vi "TagEvent.vi"(8 "error in":errorcluster, 9 "Acquisition mode in":T8, 11 "Processing loop vars in":T1 {"CurrInverter"."last updated" format="%<%H:%M\n%d/%m/%Y>T"; "CurrInverter"."set flag" items=["False", "True"]}) -> (0 "error out":errorcluster, 3 "Processing loop vars out":T1 {"CurrInverter"."last updated" format="%<%H:%M\n%d/%m/%Y>T"; "CurrInverter"."set flag" items=["False", "True"]})   [LabVIEW 2019, in "Main.lvclass"]
uses:
  Main.lvclass
  DataTypes/averaging variables.ctl
  DataTypes/ESR alarm variables.ctl
  Common/DataTypes/inverter gain range--cluster.ctl
  Common/DataTypes/inverter offset range--cluster.ctl
  Common/DataTypes/inverter info v2--cluster.ctl
  Common/DataTypes/Inverter database record v2--cluster.ctl
  DataTypes/Processing loop variables--cluster.ctl
  Common/DataTypes/Acquisition Mode--cluster.ctl
panel:
  out "Current Tag Event":i32
  out "Step Up":dbl
  out "Start time":dbl
  out "Time difference":i32
  out "Current seconds":dbl
  out "Step Down":dbl
  out "Calculated Total Power":dbl
  out "Calculated Local Power":dbl
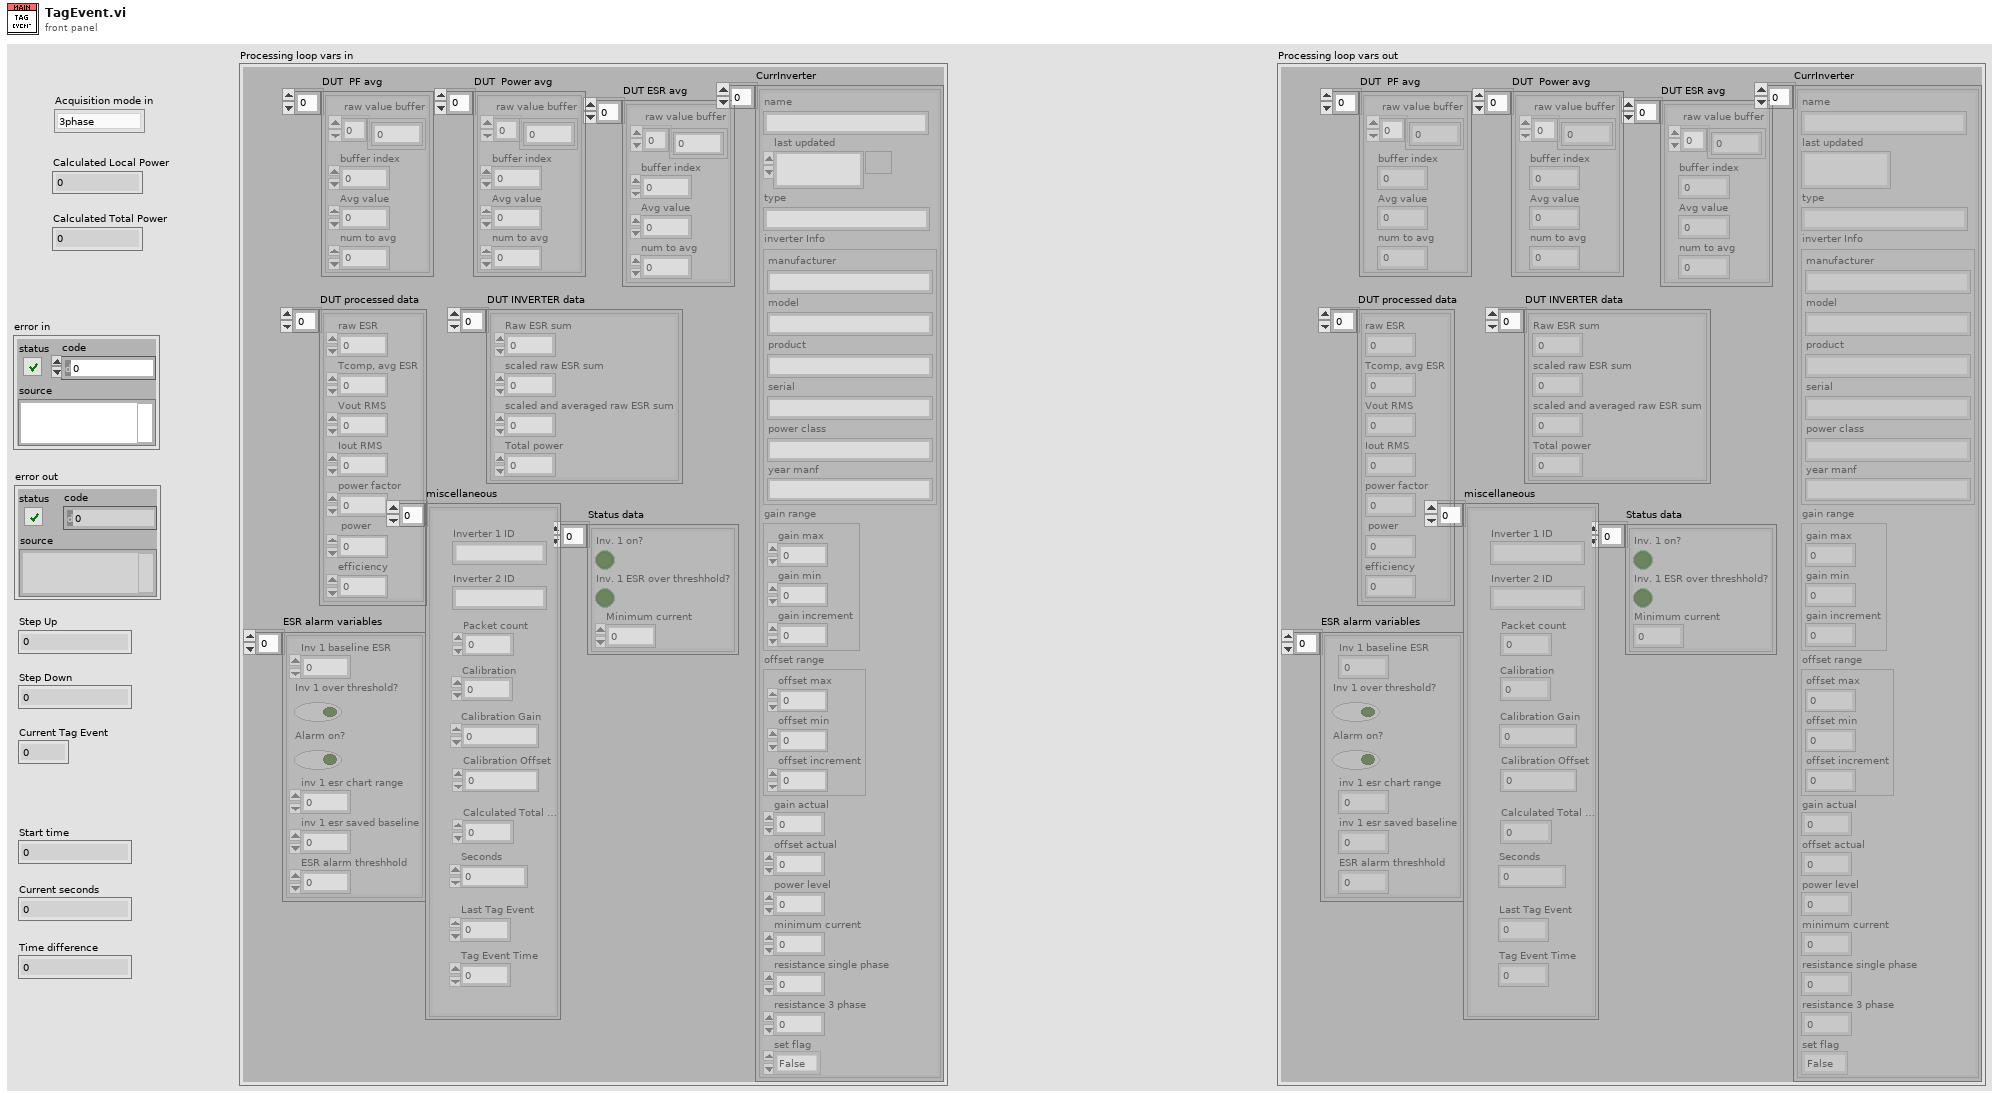
[diagram p1: front panel]
types:
  T1 = typedef "Main.lvclass/Processing loop variables--cluster.ctl" = cluster{"DUT ESR avg":T2[], "DUT  PF avg":T2[], "DUT  Power avg ":T2[], "DUT processed data":cluster{"raw ESR":dbl, "Tcomp, avg ESR":dbl, "Vout RMS":dbl, "Iout RMS":dbl, "power factor":dbl, "power":dbl, "efficiency":dbl}[], "ESR alarm variables":T3[], "Status data":cluster{"Inv. 1 on?":bool, "Inv. 1 ESR over threshhold?":bool, "Minimum current":dbl}[], "CurrInverter":T4[], "miscellaneous":cluster{"Inverter 1 ID":string, "Inverter 2 ID":string, "Packet count":u32, "Calibration":dbl, "Calibration Gain":dbl, "Calibration Offset":dbl, "Calculated Total Power":dbl, "Seconds":dbl, "Last Tag Event":dbl, "Tag Event Time":dbl}[], "DUT INVERTER data":cluster{"Raw ESR sum":dbl, "scaled raw ESR sum":dbl, "scaled and averaged raw ESR sum":dbl, "Total power":dbl}[]}
  T2 = typedef "Main.lvclass/averaging variables.ctl" = cluster{"raw value buffer":dbl[], "buffer index":i32, "Avg value":dbl, "num to avg":i32}
  T3 = typedef "Main.lvclass/ESR alarm variables.ctl" = cluster{"Inv 1 baseline ESR":dbl, "Inv 1 over threshold?":bool, "Alarm on?":bool, "inv 1 esr chart range":dbl, "inv 1 esr saved baseline":dbl, "ESR alarm threshhold":dbl}
  T4 = typedef "Inverter database record v2--cluster.ctl" = cluster{"name":string, "last updated":timestamp, "type":string, "inverter Info":T5, "gain range":T6, "offset range":T7, "gain actual":dbl, "offset actual":dbl, "power level":dbl, "minimum current":dbl, "resistance single phase":dbl, "resistance 3 phase":dbl, "set flag":u16}
  T5 = typedef "inverter info v2--cluster.ctl" = cluster{"manufacturer":string, "model":string, "product":string, "serial":string, "power class":string, "year manf":string}
  T6 = typedef "inverter gain range--cluster.ctl" = cluster{"gain max":dbl, "gain min":dbl, "gain increment":dbl}
  T7 = typedef "inverter offset range--cluster.ctl" = cluster{"offset max":dbl, "offset min":dbl, "offset increment":dbl}
  T8 = typedef "Acquisition Mode--cluster.ctl" = enum16{"3phase", "Single"}
  T9 = cluster{"raw ESR":dbl, "Tcomp, avg ESR":dbl, "Vout RMS":dbl, "Iout RMS":dbl, "power factor":dbl, "power":dbl, "efficiency":dbl}[]
  T10 = cluster{"Inverter 1 ID":string, "Inverter 2 ID":string, "Packet count":u32, "Calibration":dbl, "Calibration Gain":dbl, "Calibration Offset":dbl, "Calculated Total Power":dbl, "Seconds":dbl, "Last Tag Event":dbl, "Tag Event Time":dbl}[]
  T11 = cluster{string, "String":string, dbl, dbl, "power level":dbl, i32, "Seconds":dbl, "Iout RMS":dbl}
  T12 = cluster{"Inverter 1 ID":string, "Inverter 2 ID":string, "Packet count":u32, "Calibration":dbl, "Calibration Gain":dbl, "Calibration Offset":dbl, "Calculated Total Power":dbl, "Seconds":dbl, "Last Tag Event":dbl, "Tag Event Time":dbl}
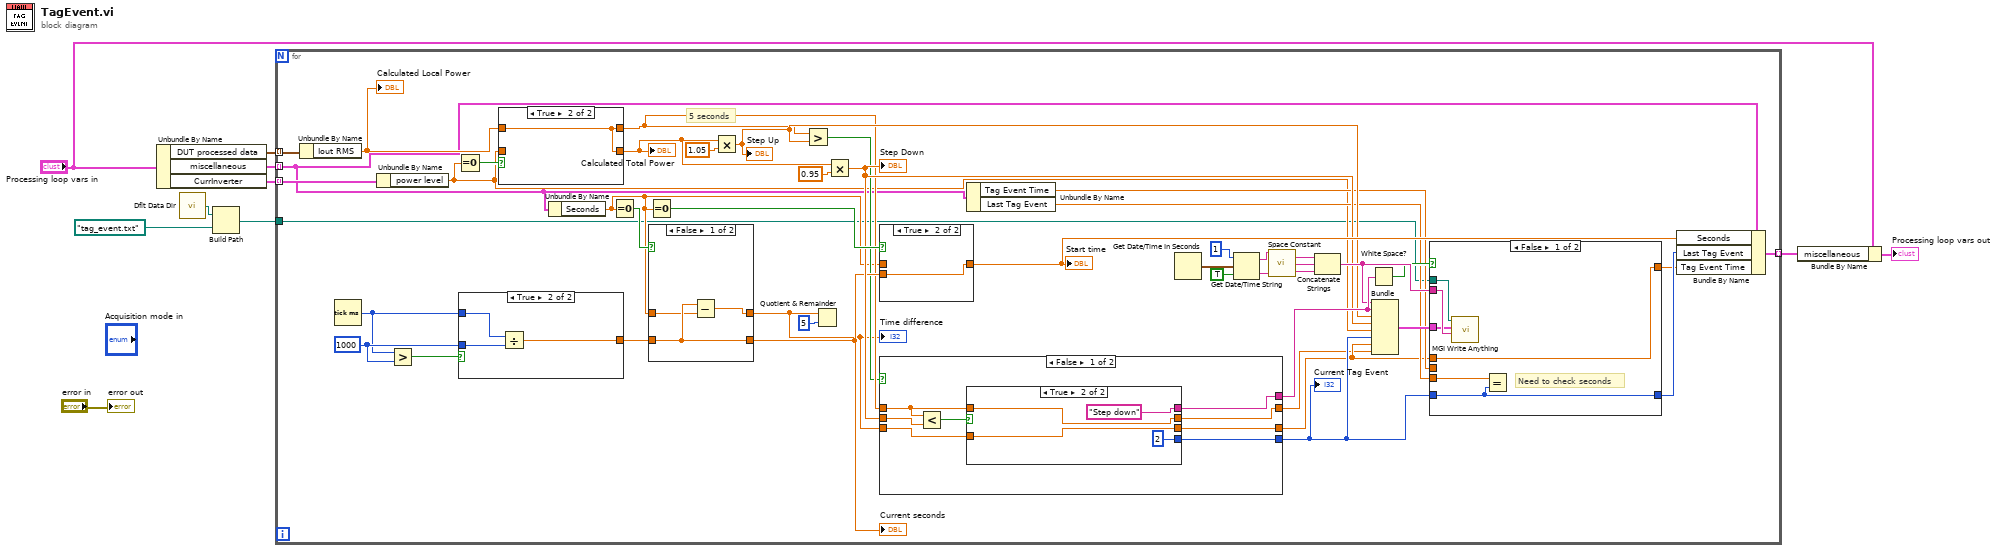
[diagram p0: block diagram]
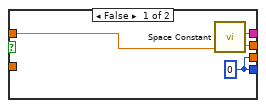
[diagram p2: hidden frame]
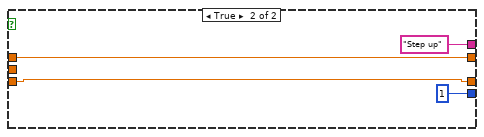
[diagram p3: hidden frame]
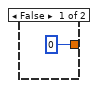
[diagram p6: hidden frame]
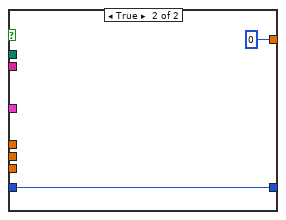
[diagram p8: hidden frame]
diagram:
  n1 = Unbundle By Name("Processing loop vars in") -> ("DUT processed data"=w10:T9, "miscellaneous"=w9:T10, "CurrInverter"=w8:T4[])
  n2 = call <vilib>:"Dflt Data Dir.vi"() -> ("App:Default Data Directory"=w3:path)
  n3 = Build Path(base path=w3, name or relative path=path "tag_event.txt") -> (appended path=w1:path)
  n4 = for {
    tunnel: w10 -> [w53] mode=indexing
    tunnel: w9 -> [w12] mode=indexing
    tunnel: w8 -> [w52] mode=indexing
    tunnel: [w13] -> w5 mode=indexing
    tunnel: w1 -> [w11]
    w41 = 1000
    # "5 seconds"
    n5 = Unbundle By Name(w53) -> ("Iout RMS"=w15:dbl)
    "Calculated Local Power" <- w15
    n6 = Tick Count (ms)() -> (millisecond timer value=w40:u32)
    n7 = Unbundle By Name(w52) -> ("power level"=w14:dbl)
    n8 = Greater?(x=w40, y=w41) -> (0:w42:bool)
    n9 = Equal To 0?(x=w14) -> (x = 0?=w36:bool)
    n10 = case shown="True" w42 {
      tunnel: w41 -> [_ w80]
      tunnel: w40 -> [_ w81]
      tunnel: [0 w79] -> w39
      frame False {
      }
      frame True {
        n11 = Divide(x=w81, y=w80) -> (x/y=w79:dbl)
      }
    }
    n12 = case shown="True" w36 {
      tunnel: w15 -> [w73 w75]
      tunnel: [w74 w75] -> w27
      tunnel: w14 -> [w74 _]
      tunnel: [w73 w75] -> w26
      frame False {
      }
      frame True {
      }
    }
    "Calculated Total Power" <- w27
    n13 = Unbundle By Name(w12) -> ("Seconds"=w16:dbl)
    n14 = Equal To 0?(x=w16) -> (x = 0?=w44:bool)
    n15 = Equal To 0?(x=w16) -> (x = 0?=w37:bool)
    n16 = case shown="False" w44 {
      tunnel: w39 -> [w84 w85]
      tunnel: [w84 w85] -> w29
      tunnel: w16 -> [w83 w86]
      tunnel: [w82 w86] -> w19
      frame False {
        n17 = Subtract(x=w84, y=w83) -> (x-y=w82:dbl)
      }
      frame True {
      }
    }
    "Current seconds" <- w29
    "Time difference" <- w19
    n18 = Multiply(x=w27, y=1.05) -> (x*y=w32:dbl)
    "Step Up" <- w32
    n19 = Greater?(x=w26, y=w32) -> (0:w25:bool)
    n20 = Quotient & Remainder(x=w19, y=5) -> ()  [unwired: 2 out]
    n21 = Multiply(x=w27, y=0.95) -> (x*y=w31:dbl)
    "Step Down" <- w31
    n22 = case shown="True" w37 {
      tunnel: w29 -> [_ w77]
      tunnel: [w76 w77] -> w38
      tunnel: w16 -> [w76 _]
      frame False {
      }
      frame True {
      }
    }
    "Start time" <- w38
    n23 = case shown="False" w25 {
      tunnel: [w61 "Step up"] -> w45
      tunnel: w26 -> [w59 w71]
      tunnel: [w58 w71] -> w17
      tunnel: w31 -> [w57 _]
      tunnel: [w56 1] -> w24
      tunnel: w19 -> [w55 w69]
      tunnel: [w54 w69] -> w18
      frame False {
        n24 = Less?(x=w59, y=w57) -> (x < y?=w60:bool)
        n25 = case shown="True" w60 {
          tunnel: [w64 "Step down"] -> w61
          tunnel: w59 -> [w63 w67]
          tunnel: [w63 w67] -> w58
          tunnel: [w62 2] -> w56
          tunnel: w55 -> [_ w65]
          tunnel: [w62 w65] -> w54
          frame False {
            w62 = 0
            n26 = call <vilib>:"Space Constant.vi"() -> ("String"=w64:string)
          }
          frame True {
          }
        }
      }
      frame True {
      }
    }
    "Current Tag Event" <- w24
    n27 = Unbundle By Name(w12) -> ("Tag Event Time"=w21:dbl, "Last Tag Event"=w20:dbl)
    n28 = Get Date/Time In Seconds() -> (seconds since 1Jan1904=w51:timestamp)
    n29 = Get Date/Time String(date format (0)=1, seconds (now)=w51, want seconds? (F)=TRUE) -> (date string=w48:string, time string=w46:string)
    n30 = call <vilib>:"Space Constant.vi"() -> ("String"=w47:string)
    n31 = Concatenate Strings(w48, w47, w46) -> (w43:string)
    n32 = White Space?(1:w45) -> (0:w30:bool)
    n33 = Bundle(w43, "String"=w45, w32, w31, "power level"=w14, w24, "Seconds"=w18, "Iout RMS"=w17) -> (w33:T11)  [unwired: 1 in]
    n34 = case shown="False" w30 {
      tunnel: w11 -> [w92 _]
      tunnel: w43 -> [w91 _]
      tunnel: w33 -> [w90 _]
      tunnel: w24 -> [w87 w94]
      tunnel: w18 -> [w89 _]
      tunnel: [w87 w94] -> w23
      tunnel: [w89 0] -> w22
      tunnel: w21 -> [_ _]
      tunnel: w20 -> [w88 _]
      frame False {
        # "Need to check seconds"
        n35 = call <userlib>:"MGI Write Anything.vi"("Section Name (Name of \"Anything\")"=w91, "Anything"=w90, "Path (dialog)"=w92) -> ()  [unwired: 6 in, 3 out]
        n36 = Equal?(x=w88, y=w87) -> ()  [unwired: 1 out]
      }
      frame True {
      }
    }
    n37 = Bundle By Name(cluster=w12, "Seconds"=w38, "Last Tag Event"=w23, "Tag Event Time"=w22) -> (w13:T12)
  }
  n38 = Bundle By Name(cluster="Processing loop vars in", "miscellaneous"=w5) -> (→"Processing loop vars out":T1)
  "error out" <- "error in"
